vi "FitSpectrum.vi"(0 "Y Values":dbl[](array[numeric]) format="%.2f", 7 "df (MHz)":dbl format="%.2f", 11 "Fit band":T2 {"center freq" format="%.2f"; "stop freq" format="%.2f"; "start" format="%.2f"}) -> (2 "stop f of fit":dbl format="%.2f", 3 "fo of fit":dbl format="%.2f", 4 "Best Linear Fit":dbl[](array[numeric]) format="%.2f", 6 "Cluster":T1 {"MSE" format="%.2f"; "pts in fit" format="%.2f"; "midband fit" format="%.2f"; "b stand dev" format="%.2f"; "intercept (b)" format="%.2f"; "m stand dev" format="%.2f"; "slope (m)" format="%.2f"}, 8 "Freq Values":dbl[](array[numeric]))   [LabVIEW 2022 SP3]
uses:
  <vilib>/Analysis/baseanly.llb/Mean (DBL).vi
  <vilib>/Analysis/NI_AALBase.lvlib
  <vilib>/Analysis/NI_AALPro.lvlib
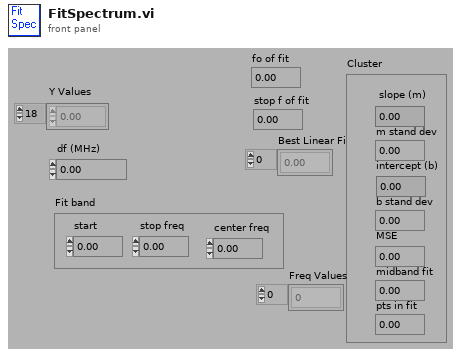
[diagram p1: front panel]
types:
  T1 = cluster{"slope (m)":dbl, "m stand dev":dbl, "intercept (b)":dbl, "b stand dev":dbl, "MSE":dbl, "midband fit":dbl, "pts in fit":dbl}
  T2 = cluster{"start":dbl, "stop freq":dbl, "center freq":dbl}
  T3 = cluster{"slope":dbl, dbl, "intercept":dbl, dbl, "residue":dbl, "f":dbl, dbl}
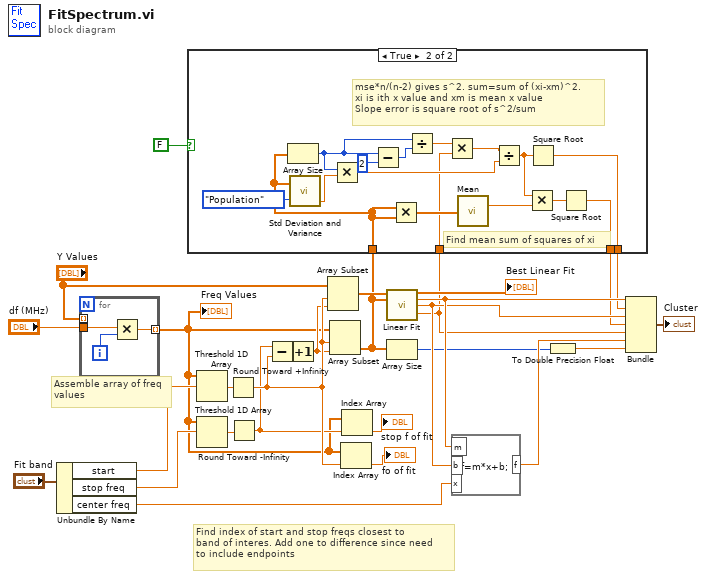
[diagram p0: block diagram]
diagram:
  # "Assemble array of freq\nvalues"
  # "Find index of start and stop freqs closest to\nband of interes. Add one to difference since need\nto include endpoints"
  n1 = Unbundle By Name("Fit band") -> ("start"=w27:dbl, "stop freq"=w26:dbl, "center freq"=w19:dbl)
  n2 = for {
    tunnel: [w30] -> w3 mode=indexing
    tunnel: "Y Values" -> [_] mode=indexing
    tunnel: "df (MHz)" -> [w29]
    i -> [w31]
    n3 = Multiply(x=w29, y=w31) -> (x*y=w30:dbl)
  }
  "Freq Values" <- w3
  n4 = Threshold 1D Array(2:w27, 3:w3) -> (0:w20:dbl)  [unwired: 1 out]
  n5 = Threshold 1D Array(2:w26, 3:w3) -> (0:w25:dbl)  [unwired: 1 out]
  n6 = Round Toward +Infinity(x=w20) -> (ceil(x): smallest int >= x=w8:dbl)
  n7 = Round Toward -Infinity(1:w25) -> (0:w6:dbl)
  n8 = Subtract(x=w6, y=w8) -> (x-y=w9:dbl)
  n9 = Increment(x=w9) -> (x+1=w7:dbl)
  n10 = Array Subset(array="Y Values", index=w8, length=w7) -> (w24:dbl[])
  n11 = Array Subset(array=w3, index=w8, length=w7) -> (w2:dbl[])
  n12 = Index Array(array=w3, index=w8) -> (element=→"fo of fit":dbl)
  n13 = Index Array(array=w3, index=w6) -> (element=→"stop f of fit":dbl)
  n14 = call <vilib>:"Linear Fit.vi"("Y"=w24, "X"=w2) -> ("Best Linear Fit"=→"Best Linear Fit":dbl[], "slope"=w18:dbl, "intercept"=w17:dbl, "residue"=w11:dbl)  [unwired: 4 in, 6 out]
  n15 = case shown="True" FALSE {
    tunnel: [_ w37] -> w16
    tunnel: [_ w36] -> w15
    tunnel: w11 -> [_ w35]
    tunnel: w2 -> [_ w34]
    frame False {
    }
    frame True {
      # "Find mean sum of squares of xi"
      # "mse*n/(n-2) gives s^2. sum=sum of (xi-xm)^2.\nxi is ith x value and xm is mean x value\nSlope error is square root of s^2/sum"
      n16 = Array Size(array=w34) -> (size(s)=w33:i32)
      n17 = call <vilib>:"Std Deviation and Variance.vi"("X"=w34, "Weighting (Sample)"=enum16{"Sample", "Population"}."Population") -> ("variance"=w47:dbl)  [unwired: 2 out]
      n18 = Multiply(x=w33, y=w47) -> (x*y=w42:dbl)
      n19 = Subtract(x=w33, y=i16 2) -> (x-y=w45:i32)
      n20 = Multiply(x=w34, y=w34) -> (x*y=w39:dbl[])
      n21 = Divide(x=w33, y=w45) -> (x/y=w44:dbl)
      n22 = Multiply(x=w44, y=w35) -> (x*y=w43:dbl)
      n23 = call-poly <vilib>:"Mean.vi"("X"=w39) -> ("mean"=w38:dbl)  [unwired: 1 out]
      n24 = Divide(x=w43, y=w42) -> (x/y=w41:dbl)
      n25 = Multiply(x=w41, y=w38) -> (x*y=w40:dbl)
      n26 = Square Root(x=w41) -> (sqrt(x)=w37:dbl)
      n27 = Square Root(x=w40) -> (sqrt(x)=w36:dbl)
    }
  }
  n28 = Array Size(array=w2) -> (size(s)=w13:i32)
  n29 = formula code="f=m*x+b;"("m"=w18, "x"=w19, "b"=w17) -> ("f"=w14:dbl)
  n30 = To Double Precision Float(number=w13) -> (double precision float=w10:dbl)
  n31 = Bundle("slope"=w18, w16, "intercept"=w17, w15, "residue"=w11, "f"=w14, w10) -> (→"Cluster":T3)  [unwired: 1 out]
